vi "PlannedPath_get.vi"(8 "error in (no error)":errorcluster) -> (0 "error out":errorcluster, 2 "PlannedPath":cluster{"X position":dbl, "Y position":dbl}[](array[cluster]))   [LabVIEW 2009, in "NetworkVarTarget.lvlib"]
uses:
  NetworkVarTarget.lvlib
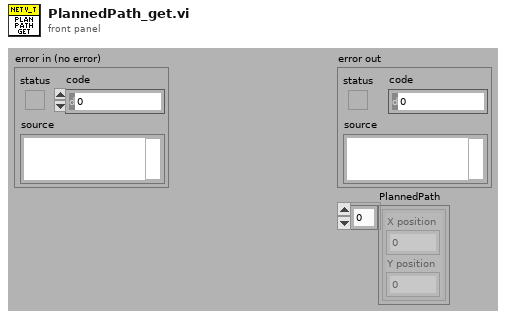
[diagram p1: front panel]
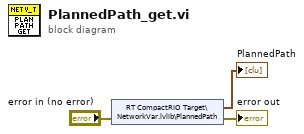
[diagram p0: block diagram]
diagram:
  n1 = shared-variable "RT CompactRIO Target\\NetworkVar.lvlib\\PlannedPath"(error in="error in (no error)") -> (→"PlannedPath":cluster{"X position":dbl, "Y position":dbl}[], error out=→"error out":errorcluster)
